vi "Check for circular references.vi"(8 "error in (no error)":errorcluster, 11 "All Variables":T1) -> (0 "error out":errorcluster, 3 "Good design":bool)   [LabVIEW 2011]
uses:
  Variable cluster.ctl
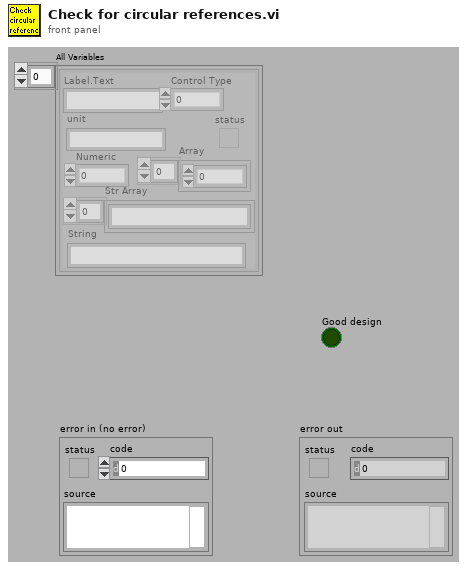
[diagram p1: front panel]
types:
  T1 = typedef "Variable cluster.ctl" = cluster{"Label.Text":string, "Control Type":u32, "Numeric":dbl, "Array":dbl[], "status":bool, "Str Array":string[], "String":string, "unit":string}[]
  T2 = cluster{"Label.Text":string, "Control Type":u32, "Numeric":dbl, "Array":dbl[], "status":bool, "Str Array":string[], "String":string, "unit":string}
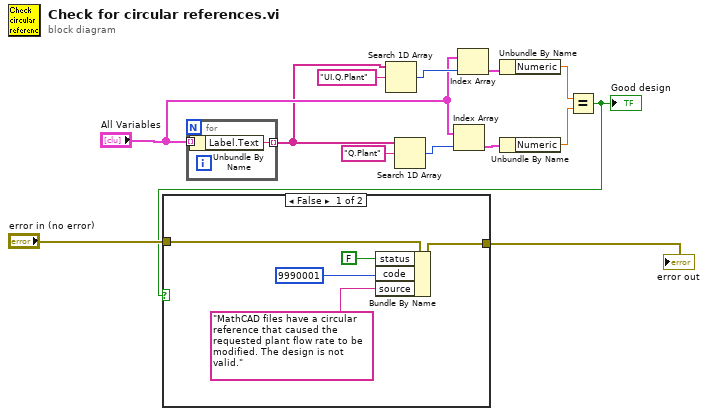
[diagram p0: block diagram]
diagram:
  n1 = for {
    tunnel: "All Variables" -> [w15] mode=indexing
    tunnel: [w14] -> w4 mode=indexing
    n2 = Unbundle By Name(w15) -> ("Label.Text"=w14:string)
  }
  n3 = Search 1D Array(1D array=w4, element="UI.Q.Plant") -> (index of element=w9:i32)  [unwired: 1 in]
  n4 = Search 1D Array(1D array=w4, element="Q.Plant") -> (index of element=w13:i32)  [unwired: 1 in]
  n5 = Index Array(array="All Variables", index=w13) -> (element=w11:T2)
  n6 = Index Array(array="All Variables", index=w9) -> (element=w7:T2)
  n7 = Unbundle By Name(w7) -> ("Numeric"=w6:dbl)
  n8 = Unbundle By Name(w11) -> ("Numeric"=w5:dbl)
  n9 = Equal?(x=w6, y=w5) -> (x = y?=w1:bool)
  "Good design" <- w1
  n10 = case shown="False" w1 {
    tunnel: "error in (no error)" -> [w20 w21]
    tunnel: [w19 w21] -> w2
    frame False {
      n11 = Bundle By Name(cluster=w20, "status"=FALSE, "code"=9990001, "source"="MathCAD files have a circular reference that caused the requested plant flow rate to be modified. The design is not valid.") -> (w19:errorcluster)
    }
    frame True {
    }
  }
  "error out" <- w2
